vi "RT Driver VI.vi"(7 "Operation":T1, 11 "Device Reference in":T2 format="%.0x") -> (0 "Error Code":i32)   [LabVIEW 2020, in "AIM ARINC 664 Engine.lvlib" / "Custom Device.lvlib"]
uses:
  Custom Device.lvlib
  <vilib>/NI/NIVS Inline Async API/_VS Inline Async API/VS Inline Async API/VS Inline Async API.lvclass
  <vilib>/NI VeriStand/Custom Device API/Custom Device API.lvlib
  Compiled.Settings.ctl
  <vilib>/NI VeriStand/Custom Device Tools/Custom Device Utility Library/Custom Device Utility Library.lvlib
  <vilib>/NI VeriStand/Custom Device API/Data Reference.ctl
  <vilib>/NI VeriStand/Custom Device API/Block Data Reference.ctl
  Inline Execution Unit Compiled Information.ctl
  Inline Execution Unit Runtime Information.ctl
  RTStateVariables.ctl
  Asynchronous Execution Unit Compiled Information.ctl
  Asynchronous Execution Unit Runtime Information.ctl
  Interfaces/Execution Unit/Execution Unit.lvclass
  Scripting/Constants.vi
  Scripting/AIM ARINC 664 Scripting.lvlib
  Interfaces/Shared Resources/Shared Resources.lvclass
  <vilib>/NI VeriStand/Custom Device API/Get Item Property (Variant).vi
  <vilib>/NI VeriStand/Custom Device API/Custom Device Item Ref.ctl
  <vilib>/NI VeriStand/Custom Device API/Hardware Interface Driver VI Operation.ctl
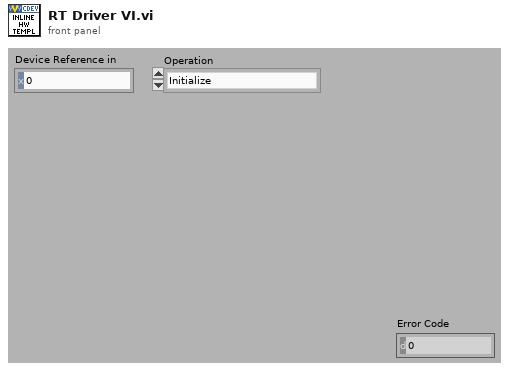
[diagram p1: front panel]
types:
  T1 = typedef "Custom Device API.lvlib/Hardware Interface Driver VI Operation.ctl" = enum16{"Initialize", "Start", "Read Data from HW", "Write Data to HW", "Close"}
  T2 = typedef "Custom Device API.lvlib/Custom Device Item Ref.ctl" = u64
  T3 = typedef "AIM ARINC 664 Engine.lvlib/Custom Device.lvlib/RTStateVariables.ctl" = cluster{"Async":refnum<class "VS Inline Async API.lvclass">, "Inline Execution Units":T4[], "Asynchronous Execution Units":T7[], "shared resources":refnum<class "Shared Resources.lvclass">}
  T4 = typedef "AIM ARINC 664 Engine.lvlib/Custom Device.lvlib/Inline Execution Unit Runtime Information.ctl" = cluster{"Execution Unit":refnum<class "Execution Unit.lvclass">, "Incoming Buffer":dbl[], "Outgoing Buffer":dbl[], "Incoming Data References":T5[], "Outgoing Data References":T6[]}
  T5 = typedef "Custom Device API.lvlib/Data Reference.ctl" = i32
  T6 = typedef "Custom Device API.lvlib/Block Data Reference.ctl" = cluster{"Data Reference":T5, "Offset":u64, "Length":u64}
  T7 = typedef "AIM ARINC 664 Engine.lvlib/Custom Device.lvlib/Asynchronous Execution Unit Runtime Information.ctl" = cluster{"Execution Unit":refnum<class "Execution Unit.lvclass">, "Incoming Channel Group Name":string, "Outgoing Channel Group Name":string, "ReadWrite Channel Group Name":string}
  T8 = typedef "AIM ARINC 664 Engine.lvlib/Custom Device.lvlib/Compiled.Settings.ctl" = cluster{"Name":string, "Inline Execution Unit Compiled Information":T9[], "Asynchronous Execution Unit Compiled Information":T10[], "Flattened Shared Resources":string}
  T9 = typedef "AIM ARINC 664 Engine.lvlib/Custom Device.lvlib/Inline Execution Unit Compiled Information.ctl" = cluster{"Flattened Execution Unit":string, "Incoming Buffer":dbl[], "Outgoing Buffer":dbl[], "Incoming Data References":T5[], "Outgoing Data References":T6[]}
  T10 = typedef "AIM ARINC 664 Engine.lvlib/Custom Device.lvlib/Asynchronous Execution Unit Compiled Information.ctl" = cluster{"Flattened Execution Unit":string, "Incoming Channel Group Name":string, "Outgoing Channel Group Name":string, "ReadWrite Channel Group Name":string}
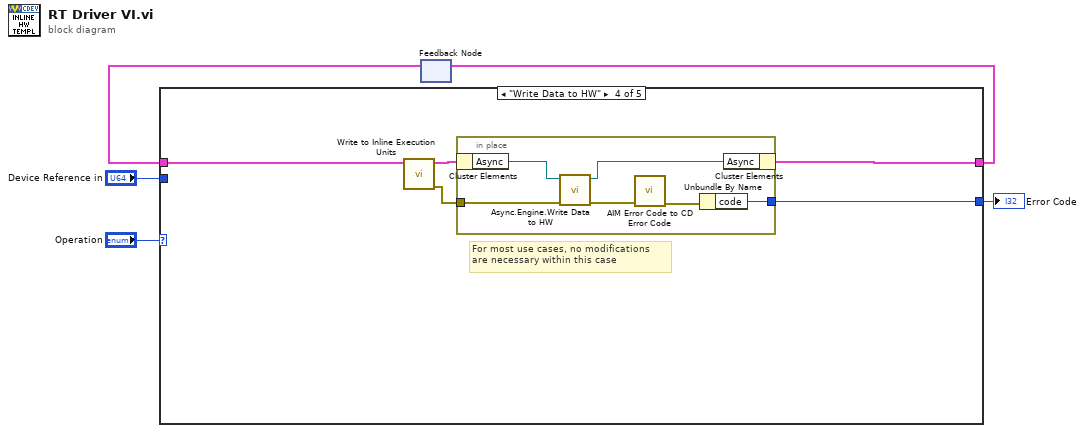
[diagram p0: block diagram]
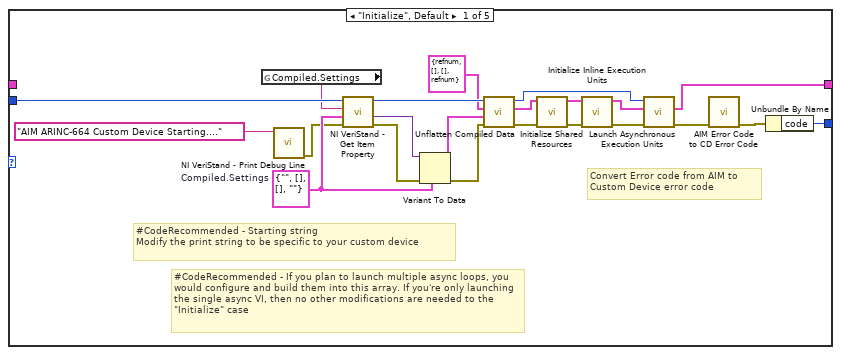
[diagram p2: hidden frame]
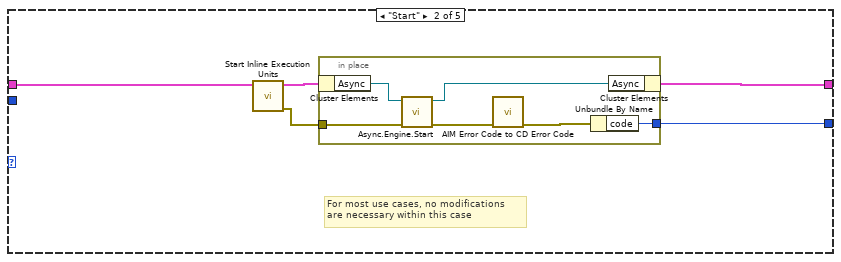
[diagram p3: hidden frame]
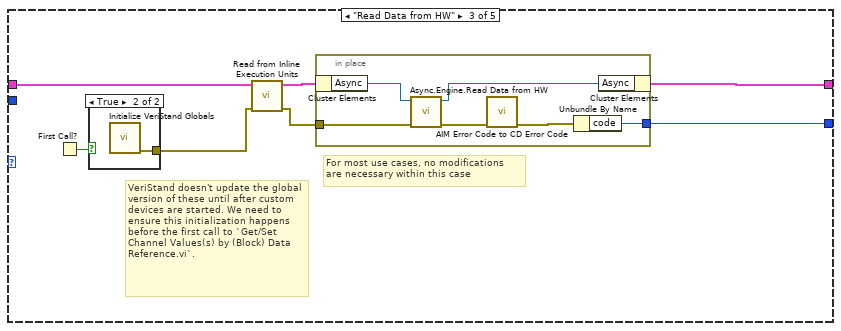
[diagram p4: hidden frame]
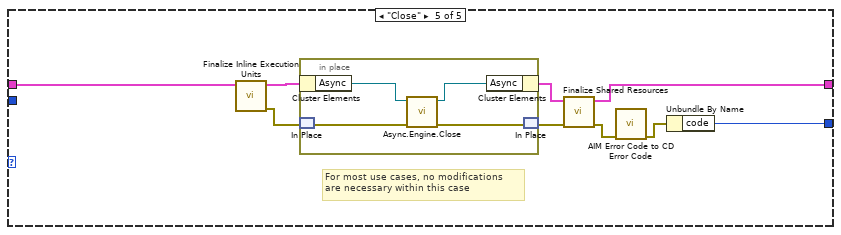
[diagram p6: hidden frame]
diagram:
  n1 = feedback #1() -> (w3:T3)  [unwired: 1 out]
  n2 = case shown="\"Write Data to HW\"" "Operation" {
    tunnel: [w16 w31 w44 w56 w66] -> w4
    tunnel: w3 -> [_ w32 w43 w55 w72]
    tunnel: "Device Reference in" -> [w26 _ _ _ _]
    tunnel: [w27 w30 w45 w57 w69] -> w1
    frame "Initialize", Default {
      w22 = T8 {"Name"="", "Inline Execution Unit Compiled Information"=[], "Asynchronous Execution Unit Compiled Information"=[], "Flattened Shared Resources"=""}  # Compiled.Settings
      # "Convert Error code from AIM to \nCustom Device error code"
      # "#CodeRecommended - Starting string\nModify the print string to be specific to your custom device"
      # "#CodeRecommended - If you plan to launch multiple async loops, you would configure and build them into this array. If you're only launching the single async VI, then no other modifications are needed to the \"Initialize\" case"
      n3 = global read "Constants.vi" "Compiled.Settings"() -> (w23:string)
      n4 = call <vilib>:"NI VeriStand - Print Debug Line.vi"("Message"="AIM ARINC-664 Custom Device Starting....") -> ("error out"=w21:errorcluster)  [unwired: 10 in]
      n5 = call-poly <vilib>:"NI VeriStand - Get Item Property.vi"("error in (no error)"=w21, "Default Value"=w22, "Property Name"=w23, "Item Ref in"=w26) -> ("error out"=w25:errorcluster, "Value"=w24:variant, "Item Ref out"=w18:T2)  [unwired: 4 in, 1 out]
      n6 = Variant To Data(error in=w25, type=w22, Variant=w24) -> (data=w19:T8, error out=w11:errorcluster)
      n7 = call "Unflatten Compiled Data.vi"("error in (no error)"=w11, "Compiled.Settings"=w19, "RTStateVariables in"=T3 {"Async"=refnum, "Inline Execution Units"=[], "Asynchronous Execution Units"=[], "shared resources"=refnum} ("RTStateVariables"), "Item Ref in"=w18) -> ("error out"=w10:errorcluster, "RTStateVariables out"=w12:T3, "Item Ref out"=w15:T2)  [unwired: 5 in]
      n8 = call "Initialize Shared Resources.vi"("error in"=w10, "RTStateVariables in"=w12) -> ("error out"=w9:errorcluster, "RTStateVariables out"=w13:T3)  [unwired: 8 in]
      n9 = call "Initialize Inline Execution Units.vi"("error in"=w9, "RTStateVariables in"=w13) -> ("error out"=w8:errorcluster, "RTStateVariables out"=w14:T3)  [unwired: 8 in]
      n10 = call "Launch Asynchronous Execution Units.vi"("error in (no error)"=w8, "RTStateVariables in"=w14, "Device Ref in"=w15) -> ("error out"=w7:errorcluster, "RTStateVariables out"=w16:T3)  [unwired: 6 in, 1 out]
      n11 = call "AIM Error Code to CD Error Code.vi"("error in"=w7) -> ("error out"=w6:errorcluster)  [unwired: 7 in, 3 out]
      n12 = Unbundle By Name(w6) -> ("code"=w27:i32)
    }
    frame "Start" {
      # "For most use cases, no modifications \nare necessary within this case"
      n13 = call "Start Inline Execution Units.vi"("RTStateVariables in"=w32) -> ("error out"=w28:errorcluster, "RTStateVariables out"=w29:T3)  [unwired: 9 in]
      n14 = in-place {
        in-place-border: [w36] -> w30
        in-place-border: w28 -> [w35]
        n15 = in-place-cluster #2(w29) -> ("Async"=w38:refnum<class "VS Inline Async API.lvclass">)
        n16 = call <vilib>:"Async.Engine.Start.vi"("error in (no error)"=w35, "VS Inline Async API in"=w38) -> ("error out"=w34:errorcluster, "VS Inline Async API out"=w37:refnum<class "VS Inline Async API.lvclass">)  [unwired: 8 in]
        n17 = call "AIM Error Code to CD Error Code.vi"("error in"=w34) -> ("error out"=w33:errorcluster)  [unwired: 7 in, 3 out]
        n18 = Unbundle By Name(w33) -> ("code"=w36:i32)
        n19 = in-place-cluster #2("Async"=w37) -> (w31:T3)
      }
    }
    frame "Read Data from HW" {
      # "VeriStand doesn't update the global version of these until after custom devices are started. We need to ensure this initialization happens before the first call to `Get/Set Channel Values(s) by (Block) Data Reference.vi`."
      # "For most use cases, no modifications \nare necessary within this case"
      n20 = First Call?() -> (First Call?: T/F=w40:bool)
      n21 = case shown="True" w40 {
        tunnel: [_ w46] -> w39
        frame False {
        }
        frame True {
          n22 = call "Initialize VeriStand Globals.vi"() -> ("error out"=w46:errorcluster)  [unwired: 11 in]
        }
      }
      n23 = call "Read from Inline Execution Units.vi"("error in (no error)"=w39, "RTStateVariables in"=w43) -> ("error out"=w41:errorcluster, "RTStateVariables out"=w42:T3)  [unwired: 8 in]
      n24 = in-place {
        in-place-border: [w50] -> w45
        in-place-border: w41 -> [w49]
        n25 = in-place-cluster #3(w42) -> ("Async"=w52:refnum<class "VS Inline Async API.lvclass">)
        n26 = call <vilib>:"Async.Engine.Read Data from HW.vi"("error in"=w49, "Async in"=w52) -> ("error out"=w48:errorcluster, "Async out"=w51:refnum<class "VS Inline Async API.lvclass">)  [unwired: 8 in]
        n27 = call "AIM Error Code to CD Error Code.vi"("error in"=w48) -> ("error out"=w47:errorcluster)  [unwired: 7 in, 3 out]
        n28 = Unbundle By Name(w47) -> ("code"=w50:i32)
        n29 = in-place-cluster #3("Async"=w51) -> (w44:T3)
      }
    }
    frame "Write Data to HW" {
      # "For most use cases, no modifications \nare necessary within this case"
      n30 = call "Write to Inline Execution Units.vi"("RTStateVariables in"=w55) -> ("error out"=w53:errorcluster, "RTStateVariables out"=w54:T3)  [unwired: 9 in]
      n31 = in-place {
        in-place-border: [w63] -> w57
        in-place-border: w53 -> [w60]
        n32 = in-place-cluster #4(w54) -> ("Async"=w62:refnum<class "VS Inline Async API.lvclass">)
        n33 = call <vilib>:"Async.Engine.Write Data to HW.vi"("error in (no error)"=w60, "VS Inline Async API in"=w62) -> ("error out"=w59:errorcluster, "VS Inline Async API out"=w61:refnum<class "VS Inline Async API.lvclass">)  [unwired: 8 in]
        n34 = call "AIM Error Code to CD Error Code.vi"("error in"=w59) -> ("error out"=w58:errorcluster)  [unwired: 7 in, 3 out]
        n35 = Unbundle By Name(w58) -> ("code"=w63:i32)
        n36 = in-place-cluster #4("Async"=w61) -> (w56:T3)
      }
    }
    frame "Close" {
      # "For most use cases, no modifications \nare necessary within this case"
      n37 = call "Finalize Inline Execution Units.vi"("RTStateVariables in"=w72) -> ("error out"=w70:errorcluster, "RTStateVariables out"=w71:T3)  [unwired: 9 in]
      n38 = in-place {
        n39 = in-place-cluster #5(w71) -> ("Async"=w76:refnum<class "VS Inline Async API.lvclass">)
        n40 = in-place-match #6(w70) -> (w74:errorcluster)
        n41 = call <vilib>:"Async.Engine.Close.vi"("error in (no error)"=w74, "Async in"=w76) -> ("error out"=w73:errorcluster, "Async out"=w75:refnum<class "VS Inline Async API.lvclass">)  [unwired: 8 in]
        n42 = in-place-cluster #5("Async"=w75) -> (w67:T3)
        n43 = in-place-match #6(w73) -> (w68:errorcluster)
      }
      n44 = call "Finalize Shared Resources.vi"("error in"=w68, "RTStateVariables in"=w67) -> ("error out"=w65:errorcluster, "RTStateVariables out"=w66:T3)  [unwired: 8 in]
      n45 = call "AIM Error Code to CD Error Code.vi"("error in"=w65) -> ("error out"=w64:errorcluster)  [unwired: 7 in, 3 out]
      n46 = Unbundle By Name(w64) -> ("code"=w69:i32)
    }
  }
  "Error Code" <- w1
  n47 = feedback-in #1(w4) -> ()
